vi "RichToFlatni_bus_monitor_api_FilterInfo.vi"(5 "OutputClusterType":T1, 11 "InputCluster":T4) -> (3 "OutputCluster":T1)   [LabVIEW 2025, in "bus_monitor_server.lvlib"]
uses:
  bus_monitor_server.lvlib
  ni_bus_monitor_api_FilterInfo.ctl
  ni_bus_monitor_api_DirectionFilter.ctl
  ni_bus_monitor_api_FrameFilter.ctl
  ni_bus_monitor_api_FilterInfo_Flat.ctl
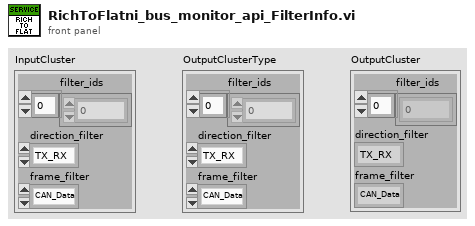
[diagram p1: front panel]
types:
  T1 = typedef "bus_monitor_server.lvlib/ni_bus_monitor_api_FilterInfo_Flat.ctl" = cluster{"filter_ids":u32[], "direction_filter":T2, "frame_filter":T3}
  T2 = typedef "bus_monitor_server.lvlib/ni_bus_monitor_api_DirectionFilter.ctl" = enum32{"TX_RX", "RX", "TX"}
  T3 = typedef "bus_monitor_server.lvlib/ni_bus_monitor_api_FrameFilter.ctl" = enum32{"CAN_Data", "CAN_Remote", "CAN_Bus_Error", "CAN_2_Data", "CAN_FD_Data", "CAN_FD_BRS_Data", "J1939_Data", "Delay", "Log_Trigger", "Start_Trigger", "All"}
  T4 = typedef "bus_monitor_server.lvlib/ni_bus_monitor_api_FilterInfo.ctl" = cluster{"filter_ids":u32[], "direction_filter":T2, "frame_filter":T3}
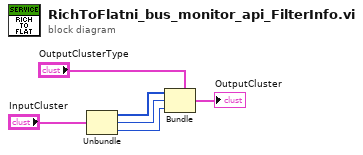
[diagram p0: block diagram]
diagram:
  n1 = Unbundle "Unbundle"("InputCluster") -> ("filter_ids"=w3:u32[], "direction_filter"=w2:T2, "frame_filter"=w1:T3)
  n2 = Bundle "Bundle"(cluster="OutputClusterType", "filter_ids"=w3, "direction_filter"=w2, "frame_filter"=w1) -> (→"OutputCluster":T1)
